vi "Flatten XML String.vi"(6 "Include Type Attribute (T)":bool=TRUE, 7 "Root ID":string, 8 "Error In":errorcluster, 11 "Tree":T1) -> (0 "Error Out":errorcluster, 1 "XML String":string, 3 "Tree":T1)   [LabVIEW 2020, in "NI_VIAnCFGDataStructure.lvlib" / "Tree.lvclass"]
doc: "Flatten the specified Tree to XML representation. Any existing Tree can be used as the Root element in XML representation. This method can be used to copy contents of one Tree Manager to another.\n\n<b>WARNING</b> This methods implements basic LV implementaion for parsing the XML. It is supported on multiple targets because it does not use the native LV DOM parser. This means it might be less optimal and not handle all XML parsing errors. Please test it extensively before using in your final design.\n\n<b>WARNING</b> All Tree names that contain a space character will have it replaced by underscore character. This is required by XML specification."
uses:
  <vilib>/addons/analyzer/VIAnCFGDataStructure/Tree Manager/Tree.lvclass
  <vilib>/addons/analyzer/VIAnCFGDataStructure/Tree Manager/Typedefs/Session Handle.ctl
  <vilib>/addons/analyzer/VIAnCFGDataStructure/Tree Manager/Tree.lvclass/Tree.ctl
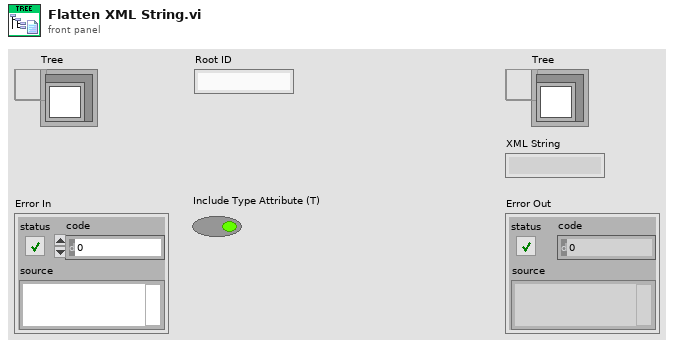
[diagram p1: front panel]
types:
  T1 = typedef "NI_VIAnCFGDataStructure.lvlib/Tree.lvclass/Session Handle.ctl" = refnum<data-value>
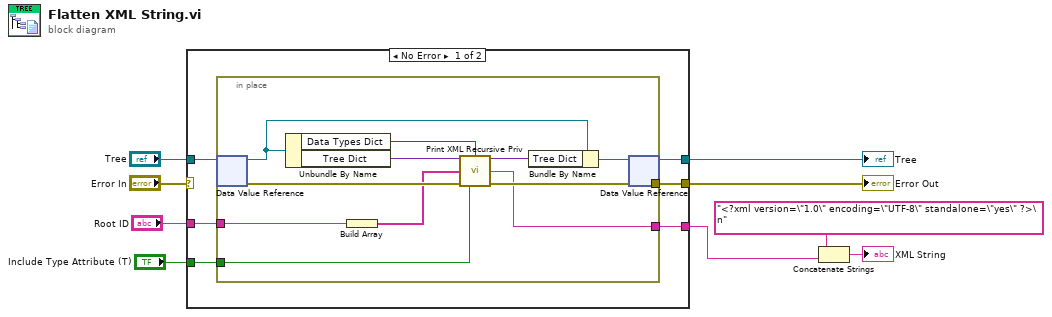
[diagram p0: block diagram]
diagram:
  n1 = case shown="No Error" "Error In" {
    selector: "Error In" -> [_ w27]
    tunnel: "Tree" -> [w15 w28]
    tunnel: [w14 w28] -> w8
    tunnel: [w13 w27] -> w6
    tunnel: "Root ID" -> [w12 _]
    tunnel: [w11 _] -> w2
    tunnel: "Include Type Attribute (T)" -> [w10 _]
    frame No Error {
      n2 = in-place {
        in-place-border: [w25] -> w13
        in-place-border: w12 -> [w22]
        in-place-border: [w21] -> w11
        in-place-border: w10 -> [w16]
        n3 = in-place-dvr #1(w15) -> (w26:refnum<class "Tree.lvclass">, w23:errorcluster)
        n4 = Unbundle By Name(w26) -> ("Data Types Dict"=w17:variant, "Tree Dict"=w20:variant)
        n5 = Build Array(w22) -> (w18:string[])
        n6 = call <vilib>:"Print XML Recursive Priv.vi"("Tree Dictionary In"=w20, "Data Types Dict"=w17, "Child IDs"=w18, "error in"=w23, "Include Type Attribute"=w16) -> ("Tree Dictionary Out"=w19:variant, "XML String"=w21:string, "error out"=w25:errorcluster)  [unwired: 8 in]
        n7 = Bundle By Name(cluster=w26, "Tree Dict"=w19) -> (w24:refnum<class "Tree.lvclass">)
        n8 = in-place-dvr #1(w24) -> (w14:T1)  [unwired: 1 out]
      }
    }
    frame Error {
    }
  }
  "Tree" <- w8
  "Error Out" <- w6
  n9 = Concatenate Strings("<?xml version=\"1.0\" encoding=\"UTF-8\" standalone=\"yes\" ?>\n", w2) -> (→"XML String":string)
